vi "Initialize Connection with CD.vi"(8 "error in (no error)":errorcluster, 10 "TCP Service":string, 11 "IP Address":string) -> (0 "error out":errorcluster, 3 "connection info out":T1)   [LabVIEW 2018, in "Instrument Host Automation API.lvlib"]
uses:
  Instrument Host Automation API.lvlib
  <vilib>/NI/STM/NI STM.lvlib
  <vilib>/NI/STM/TCP/Write Meta Data (TCP Ref).vi
  <vilib>/NI/STM/SubVIs/MetaDataElement.ctl
  <vilib>/NI/STM/TCP/TCP Connection Info.ctl
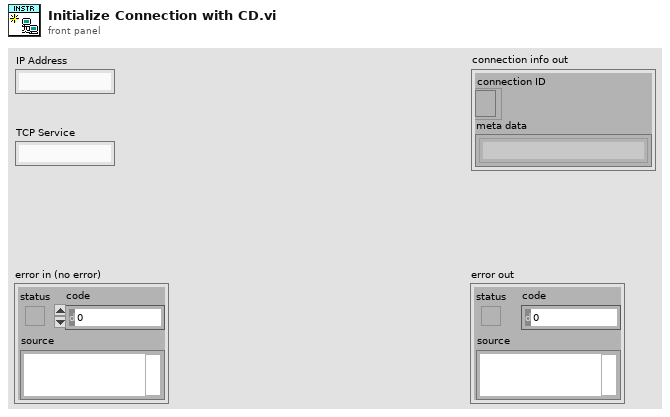
[diagram p1: front panel]
types:
  T1 = typedef "NI STM.lvlib/TCP Connection Info.ctl" = cluster{"connection ID":refnum<k5>, "meta data":T2[]}
  T2 = typedef "NI STM.lvlib/MetaDataElement.ctl" = string
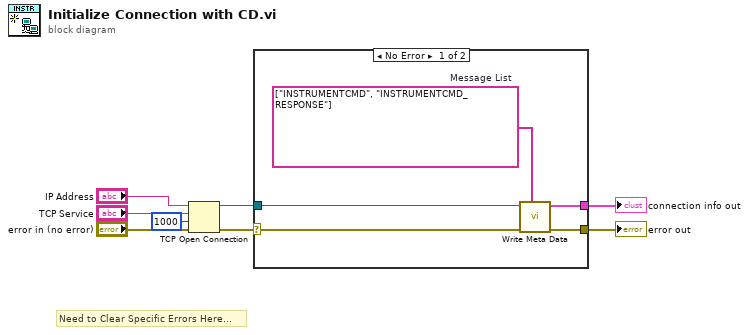
[diagram p0: block diagram]
diagram:
  # "Need to Clear Specific Errors Here..."
  n1 = TCP Open Connection(address="IP Address", remote port or service name="TCP Service", timeout ms (60000)=1000, error in (no error)="error in (no error)") -> (connection ID=w8:refnum<k5>, error out=w7:errorcluster)  [unwired: 1 in]
  n2 = case shown="No Error" w7 {
    selector: w7 -> [w10 w14]
    tunnel: w8 -> [w12 _]
    tunnel: [w11 w14] -> w1
    tunnel: [w9 _] -> w5
    frame No Error {
      w13 = string[] ["INSTRUMENTCMD", "INSTRUMENTCMD_RESPONSE"]  # Message List
      n3 = call-poly <vilib>:"Write Meta Data.vi"("meta data"=w13, "error in"=w10, "connection ID"=w12) -> ("error out"=w11:errorcluster, "connection info out"=w9:T1)  [unwired: 7 in]
    }
    frame Error {
    }
  }
  "error out" <- w1
  "connection info out" <- w5
